vi "Create Events Table_Beltwatch.vi"() -> ()   [LabVIEW 2017, in "Copy of Beltwatch SQLite.lvlib"]
uses:
  Database/Copy of Beltwatch SQLite.lvlib
  Common64/Database/SQ Lite/SQ Lite Cluster Action.ctl
  Beltwatch/SourceCode/BeltWatch Event.ctl
  Beltwatch/SourceCode/BeltWatch Event type.ctl
  Beltwatch/SourceCode/BeltWatch Reading.ctl
  Beltwatch/SourceCode/BeltWatch Alarm Priority.ctl
  Beltwatch/SourceCode/BeltWatch 2D overlay.ctl
  Beltwatch/SourceCode/Overlay mode.ctl
  Beltwatch/SourceCode/Events class.ctl
panel:
  in  "Event":T1={"Position"=17279.321740347055, "Event Type"=enum."Splice", "Area"=261.6138488586849, "Channels"=4503599627369984, "Start position"=17276.619140625, "End  position"=17282.02434006911, "Name"="", "Offset"=0.0, "Length"=1987.8302132084298, "Action marker"="", "Event"=array672x65[43680 elements], "# Defects"=137, "jpg Image"="ASD", "chan maxs"=[0.0, 0.0, 0.0, 0.0, 0.0, 0.0, 0.0, 0.0, 0.0, 0.768, 1.157, 1.845, 4.443, 7.03, 7.383, 6.949, 6.966, 7.121, 6.212, 5.231, 4.772, 4.836, 4.757, 4.587, 4.548, 4.517, 4.666, 4.782, 5.001, 5.174, 5.371, 5.176, 5.098, 4.922, 4.915, 4.636, 4.584, 4.794, 4.884, 4.908, 4.821, 5.046, 5.03, 5.533, 6.356, 7.56, 5.75, 5.5, 7.87, 6.962, 6.495, 1.517, 0.0, 0.0, 0.0, 0.0, 0.0, 0.0, 0.0, 0.0, 0.0, 0.0, 0.0, 0.0], "chan mins"=[0.0, 0.0, 0.0, 0.0, 0.0, 0.0, 0.0, 0.0, 0.0, -1.193, -1.906, -3.257, -6.752, -6.705, -5.152, -4.988, -4.848, -4.552, -4.04, -3.624, -3.41, -3.38, -3.179, -3.134, -3.041, -3.144, -3.022, -3.138, -3.276, -3.433, -3.191, -3.066, -3.021, -2.965, -2.907, -2.884, -2.847, -3.026, -3.293, -3.238, -3.475, -3.528, -3.781, -3.92, -4.795, -6.373, -3.84, -4.344, -6.783, -6.818, -6.448, -1.468, 0.0, 0.0, 0.0, 0.0, 0.0, 0.0, 0.0, 0.0, 0.0, 0.0, 0.0, 0.0], "TimeStamp"=3620638606.9, "Readings"=[{"Reading #"=0, "Readings"=[3.9289019107818604], "Reading Name"="Splice distortion", "Type"=enum."Defect", "Alarm priority"=enum."No Alarm", "Display precision"=0}, {"Reading #"=1, "Readings"=[1328.95654296875], "Reading Name"="Splice length", "Type"=enum."Defect", "Alarm priority"=enum."No Alarm", "Display precision"=0}, {"Reading #"=2, "Readings"=[0.0], "Reading Name"="Splice necking", "Type"=enum."Defect", "Alarm priority"=enum."No Alarm", "Display precision"=0}, {"Reading #"=3, "Readings"=[0.0], "Reading Name"="Splice Max Amplitude ", "Type"=enum."Defect", "Alarm priority"=enum."No Alarm", "Display precision"=0}, {"Reading #"=4, "Readings"=[0.0], "Reading Name"="Width at Splice", "Type"=enum."Defect", "Alarm priority"=enum."No Alarm", "Display precision"=0}, {"Reading #"=5, "Readings"=[0.0], "Reading Name"="Tracking at splice", "Type"=enum."Defect", "Alarm priority"=enum."No Alarm", "Display precision"=0}, {"Reading #"=0, "Readings"=[2.0], "Reading Name"="No. Breaks", "Type"=enum."Defect", "Alarm priority"=enum."No Alarm", "Display precision"=0}, {"Reading #"=1, "Readings"=[7.372896194458008], "Reading Name"="Max  Amplitude (V)", "Type"=enum."Defect", "Alarm priority"=enum."No Alarm", "Display precision"=0}, {"Reading #"=2, "Readings"=[10.810811042785645], "Reading Name"="% Belt Width", "Type"=enum."Defect", "Alarm priority"=enum."No Alarm", "Display precision"=0}, {"Reading #"=3, "Readings"=[0.0], "Reading Name"="% Center Width (%)", "Type"=enum."Defect", "Alarm priority"=enum."No Alarm", "Display precision"=0}, {"Reading #"=4, "Readings"=[0.0], "Reading Name"=" % Max Edge Width", "Type"=enum."Defect", "Alarm priority"=enum."No Alarm", "Display precision"=0}], "ID"=2754970069, "New"=FALSE, "Hires Track"=array672x3[2016 elements], "2D overlay"=[{"group"=[{"X Out"=[1.1431535, 1.1364423, 1.127946, 1.1181517, 1.1072357, 1.0956326, 1.0842199, 1.0731843, 1.0618212, 1.0499833, 1.0380819, 1.0261621, 1.0141459, 1.0021335, 0.990249, 0.9785226, 0.9667934, 0.9549859, 0.9433727, 0.9321445, 0.9210712, 0.909718, 0.8976863, 0.8850422, 0.8726231, 0.8613366, 0.85129416, 0.84175557, 0.8317911, 0.82107306, 0.80985045, 0.79857224, 0.7876048, 0.77725023, 0.76879144, 0.76415265, 0.7633842, 0.7641389, 0.7641741], "Y Out"=[0.40625, 0.4375, 0.46875, 0.5, 0.53125, 0.5625, 0.59375, 0.625, 0.65625, 0.6875, 0.71875, 0.75, 0.78125, 0.8125, 0.84375, 0.875, 0.90625, 0.9375, 0.96875, 1.0, 1.03125, 1.0625, 1.09375, 1.125, 1.15625, 1.1875, 1.21875, 1.25, 1.28125, 1.3125, 1.34375, 1.375, 1.40625, 1.4375, 1.46875, 1.5, 1.53125, 1.5625, 1.59375]}], "Color "=16711680, "Mode"=enum."Line"}, {"group"=[{"X Out"=[1.144922, 1.1339688, 1.1230156, 1.1120626, 1.1011094, 1.0901562, 1.0792031, 1.06825, 1.0572968, 1.0463436, 1.0353905, 1.0244373, 1.0134841, 1.002531, 0.99157786, 0.98062474, 0.96967155, 0.9587184, 0.94776523, 0.9368121, 0.925859, 0.9149058, 0.90395266, 0.89299953, 0.88204634, 0.8710932, 0.86014, 0.8491869, 0.83823377, 0.8272806, 0.81632745, 0.80537426, 0.79442114, 0.783468, 0.7725148, 0.7615617, 0.75060856, 0.7396554, 0.72870225], "Y Out"=[0.40625, 0.4375, 0.46875, 0.5, 0.53125, 0.5625, 0.59375, 0.625, 0.65625, 0.6875, 0.71875, 0.75, 0.78125, 0.8125, 0.84375, 0.875, 0.90625, 0.9375, 0.96875, 1.0, 1.03125, 1.0625, 1.09375, 1.125, 1.15625, 1.1875, 1.21875, 1.25, 1.28125, 1.3125, 1.34375, 1.375, 1.40625, 1.4375, 1.46875, 1.5, 1.53125, 1.5625, 1.59375]}], "Color "=6618880, "Mode"=enum."Line"}, {"group"=[{"X Out"=[1.8756652, 1.8688927, 1.859341, 1.848455, 1.838679, 1.8297793, 1.8196244, 1.8080461, 1.7966759, 1.7862864, 1.7759557, 1.7647399, 1.7527764, 1.7405266, 1.7283434, 1.7166883, 1.7059686, 1.6960664, 1.686259, 1.6760231, 1.6652597, 1.6537125, 1.6410868, 1.627567, 1.6140205, 1.6013763, 1.5898267, 1.5787398, 1.5671003, 1.5549228, 1.5439305, 1.535136, 1.5267466, 1.5169554, 1.507604, 1.5030762, 1.5055563, 1.5104653, 1.5101554], "Y Out"=[0.40625, 0.4375, 0.46875, 0.5, 0.53125, 0.5625, 0.59375, 0.625, 0.65625, 0.6875, 0.71875, 0.75, 0.78125, 0.8125, 0.84375, 0.875, 0.90625, 0.9375, 0.96875, 1.0, 1.03125, 1.0625, 1.09375, 1.125, 1.15625, 1.1875, 1.21875, 1.25, 1.28125, 1.3125, 1.34375, 1.375, 1.40625, 1.4375, 1.46875, 1.5, 1.53125, 1.5625, 1.59375]}], "Color "=16711680, "Mode"=enum."Line"}, {"group"=[{"X Out"=[1.8790404, 1.8683056, 1.8575706, 1.8468357, 1.8361009, 1.825366, 1.8146311, 1.8038963, 1.7931614, 1.7824265, 1.7716916, 1.7609568, 1.7502218, 1.7394869, 1.7287521, 1.7180172, 1.7072823, 1.6965475, 1.6858126, 1.6750777, 1.6643429, 1.653608, 1.642873, 1.6321381, 1.6214033, 1.6106684, 1.5999335, 1.5891987, 1.5784638, 1.5677289, 1.5569941, 1.5462592, 1.5355242, 1.5247893, 1.5140545, 1.5033196, 1.4925847, 1.4818499, 1.471115], "Y Out"=[0.40625, 0.4375, 0.46875, 0.5, 0.53125, 0.5625, 0.59375, 0.625, 0.65625, 0.6875, 0.71875, 0.75, 0.78125, 0.8125, 0.84375, 0.875, 0.90625, 0.9375, 0.96875, 1.0, 1.03125, 1.0625, 1.09375, 1.125, 1.15625, 1.1875, 1.21875, 1.25, 1.28125, 1.3125, 1.34375, 1.375, 1.40625, 1.4375, 1.46875, 1.5, 1.53125, 1.5625, 1.59375]}], "Color "=6618880, "Mode"=enum."Line"}, {"group"=[{"X Out"=[2.474482, 2.4683018, 2.4580495, 2.4460716, 2.4337676, 2.4210174, 2.4081779, 2.3957546, 2.3835855, 2.371664, 2.360103, 2.3485243, 2.3367019, 2.32491, 2.3134542, 2.3026762, 2.2927556, 2.2830057, 2.2726293, 2.262022, 2.2517924, 2.2415245, 2.2306695, 2.2193754, 2.2081182, 2.197146, 2.1865563, 2.1765766, 2.1669314, 2.156789, 2.1457903, 2.1341538, 2.1224358, 2.1115074, 2.1018374, 2.0934274, 2.0864358, 2.080968, 2.0776985, 2.078398], "Y Out"=[0.375, 0.40625, 0.4375, 0.46875, 0.5, 0.53125, 0.5625, 0.59375, 0.625, 0.65625, 0.6875, 0.71875, 0.75, 0.78125, 0.8125, 0.84375, 0.875, 0.90625, 0.9375, 0.96875, 1.0, 1.03125, 1.0625, 1.09375, 1.125, 1.15625, 1.1875, 1.21875, 1.25, 1.28125, 1.3125, 1.34375, 1.375, 1.40625, 1.4375, 1.46875, 1.5, 1.53125, 1.5625, 1.59375]}], "Color "=16711680, "Mode"=enum."Line"}, {"group"=[{"X Out"=[2.4696484, 2.4589303, 2.4482121, 2.437494, 2.4267757, 2.4160576, 2.4053395, 2.3946214, 2.3839033, 2.3731852, 2.362467, 2.351749, 2.3410306, 2.3303125, 2.3195944, 2.3088763, 2.2981582, 2.28744, 2.276722, 2.2660036, 2.2552855, 2.2445674, 2.2338493, 2.2231312, 2.212413, 2.201695, 2.1909766, 2.1802585, 2.1695404, 2.1588223, 2.1481042, 2.137386, 2.126668, 2.1159499, 2.1052315, 2.0945134, 2.0837953, 2.0730772, 2.062359, 2.051641], "Y Out"=[0.375, 0.40625, 0.4375, 0.46875, 0.5, 0.53125, 0.5625, 0.59375, 0.625, 0.65625, 0.6875, 0.71875, 0.75, 0.78125, 0.8125, 0.84375, 0.875, 0.90625, 0.9375, 0.96875, 1.0, 1.03125, 1.0625, 1.09375, 1.125, 1.15625, 1.1875, 1.21875, 1.25, 1.28125, 1.3125, 1.34375, 1.375, 1.40625, 1.4375, 1.46875, 1.5, 1.53125, 1.5625, 1.59375]}], "Color "=6618880, "Mode"=enum."Line"}, {"group"=[{"X Out"=[1.7447797, 1.7451751, 1.741319, 1.7346371, 1.7244854, 1.7100781, 1.6942157, 1.6798319, 1.6669112, 1.6542252, 1.6415849, 1.6298665, 1.6191487, 1.6083951, 1.5975679, 1.5876111, 1.5781267, 1.5678036, 1.5566093, 1.5451726, 1.5332894, 1.5207548, 1.5084059, 1.4974245, 1.4880521, 1.4792299, 1.4697143, 1.4593418, 1.4490005, 1.4395406, 1.4302719, 1.418966, 1.4053056, 1.3919517, 1.3801312, 1.369776, 1.3635503, 1.3650829], "Y Out"=[0.40625, 0.4375, 0.46875, 0.5, 0.53125, 0.5625, 0.59375, 0.625, 0.65625, 0.6875, 0.71875, 0.75, 0.78125, 0.8125, 0.84375, 0.875, 0.90625, 0.9375, 0.96875, 1.0, 1.03125, 1.0625, 1.09375, 1.125, 1.15625, 1.1875, 1.21875, 1.25, 1.28125, 1.3125, 1.34375, 1.375, 1.40625, 1.4375, 1.46875, 1.5, 1.53125, 1.5625]}], "Color "=16711680, "Mode"=enum."Line"}, {"group"=[{"X Out"=[1.7556474, 1.7446698, 1.7336922, 1.7227145, 1.7117369, 1.7007593, 1.6897817, 1.678804, 1.6678264, 1.6568488, 1.6458712, 1.6348935, 1.6239159, 1.6129383, 1.6019607, 1.590983, 1.5800055, 1.5690279, 1.5580503, 1.5470726, 1.536095, 1.5251174, 1.5141398, 1.5031621, 1.4921845, 1.4812069, 1.4702293, 1.4592516, 1.448274, 1.4372964, 1.4263188, 1.4153411, 1.4043636, 1.393386, 1.3824084, 1.3714308, 1.3604531, 1.3494755], "Y Out"=[0.40625, 0.4375, 0.46875, 0.5, 0.53125, 0.5625, 0.59375, 0.625, 0.65625, 0.6875, 0.71875, 0.75, 0.78125, 0.8125, 0.84375, 0.875, 0.90625, 0.9375, 0.96875, 1.0, 1.03125, 1.0625, 1.09375, 1.125, 1.15625, 1.1875, 1.21875, 1.25, 1.28125, 1.3125, 1.34375, 1.375, 1.40625, 1.4375, 1.46875, 1.5, 1.53125, 1.5625]}], "Color "=6618880, "Mode"=enum."Line"}, {"group"=[{"X Out"=[4.364139, 4.46226, 4.364139, 4.46226], "Y Out"=[1.384375, 1.384375, 1.446875, 1.446875]}], "Color "=16727850, "Mode"=enum."Oval"}, {"group"=[{"X Out"=[2.1874433, 2.1874433, 2.1874433, 2.1874433], "Y Out"=[1.5, 1.5, 1.53125, 1.53125]}], "Color "=16727850, "Mode"=enum."Oval"}], "update"=FALSE, "Field #"=0, "Events Class"=enum."Reference", "Sync"=FALSE, "Insert Offset"=0.0, "Next trend"=0.0, "Speed"=0.0}
  out "source":string
  in  "Pre String":string="DROP TABLE IF EXISTS events;\n\n\nCREATE TABLE events (\n  db_id INTEGER PRIMARY KEY AUTOINCREMENT"
  in  "Readingse":T8[](array[typedef])=[{"Include"=TRUE, "Name"="Reading #", "SQLite3 type"=enum."SQLITE_INTEGER"}, {"Include"=TRUE, "Name"="Readings", "SQLite3 type"=enum."SQLITE3_TEXT"}, {"Include"=TRUE, "Name"="Reading Name", "SQLite3 type"=enum."SQLITE3_TEXT"}, {"Include"=TRUE, "Name"="TypeVal", "SQLite3 type"=enum."SQLITE_INTEGER"}, {"Include"=TRUE, "Name"="Alarm priority", "SQLite3 type"=enum."SQLITE_INTEGER"}, {"Include"=FALSE, "Name"="Display precision", "SQLite3 type"=enum."undefined type (0)"}, {"Include"=TRUE, "Name"="TypeStr", "SQLite3 type"=enum."SQLITE3_TEXT"}, {"Include"=TRUE, "Name"="AlarmPriorityStr", "SQLite3 type"=enum."SQLITE3_TEXT"}]
  out "?":errorcluster
  out "String":string
  out "SQLite3 type":T9(ring)
  in  "Events":T8[](array[typedef])=[{"Include"=TRUE, "Name"="Position", "SQLite3 type"=enum."SQLITE_INTEGER"}, {"Include"=TRUE, "Name"="Event Type", "SQLite3 type"=enum."SQLITE_INTEGER"}, {"Include"=TRUE, "Name"="Area", "SQLite3 type"=enum."SQLITE_INTEGER"}, {"Include"=TRUE, "Name"="Channels", "SQLite3 type"=enum."SQLITE_INTEGER"}, {"Include"=TRUE, "Name"="Start position", "SQLite3 type"=enum."SQLITE_INTEGER"}, {"Include"=TRUE, "Name"="End  position", "SQLite3 type"=enum."SQLITE_INTEGER"}, {"Include"=TRUE, "Name"="Name", "SQLite3 type"=enum."SQLITE3_TEXT"}, {"Include"=TRUE, "Name"="Offset", "SQLite3 type"=enum."SQLITE_INTEGER"}, {"Include"=TRUE, "Name"="Length", "SQLite3 type"=enum."SQLITE_INTEGER"}, {"Include"=TRUE, "Name"="Action marker", "SQLite3 type"=enum."SQLITE3_TEXT"}, {"Include"=FALSE, "Name"="Event", "SQLite3 type"=enum."SQLITE_INTEGER"}, {"Include"=TRUE, "Name"="# Defects", "SQLite3 type"=enum."SQLITE_INTEGER"}, {"Include"=TRUE, "Name"="jpg Image", "SQLite3 type"=enum."SQLITE_BLOB"}, {"Include"=FALSE, "Name"="chan maxs", "SQLite3 type"=enum."SQLITE_INTEGER"}, {"Include"=FALSE, "Name"="chan mins", "SQLite3 type"=enum."SQLITE_INTEGER"}, {"Include"=TRUE, "Name"="TimeStamp", "SQLite3 type"=enum."SQLITE_INTEGER"}, {"Include"=TRUE, "Name"="Readings", "SQLite3 type"=enum."SQLITE_INTEGER"}, {"Include"=TRUE, "Name"="ID", "SQLite3 type"=enum."SQLITE_INTEGER"}, {"Include"=TRUE, "Name"="New", "SQLite3 type"=enum."SQLITE_INTEGER"}, {"Include"=TRUE, "Name"="Hires Track", "SQLite3 type"=enum."SQLITE_INTEGER"}, {"Include"=FALSE, "Name"="2D overlay", "SQLite3 type"=enum."SQLITE_INTEGER"}, {"Include"=FALSE, "Name"="update", "SQLite3 type"=enum."SQLITE_INTEGER"}, {"Include"=TRUE, "Name"="Field #", "SQLite3 type"=enum."SQLITE_INTEGER"}, {"Include"=TRUE, "Name"="Events Class", "SQLite3 type"=enum."SQLITE_INTEGER"}, {"Include"=TRUE, "Name"="Sync", "SQLite3 type"=enum."SQLITE_INTEGER"}, {"Include"=TRUE, "Name"="Insert Offset", "SQLite3 type"=enum."SQLITE_INTEGER"}, {"Include"=TRUE, "Name"="Next trend", "SQLite3 type"=enum."SQLITE_INTEGER"}, {"Include"=TRUE, "Name"="Speed", "SQLite3 type"=enum."SQLITE_INTEGER"}]
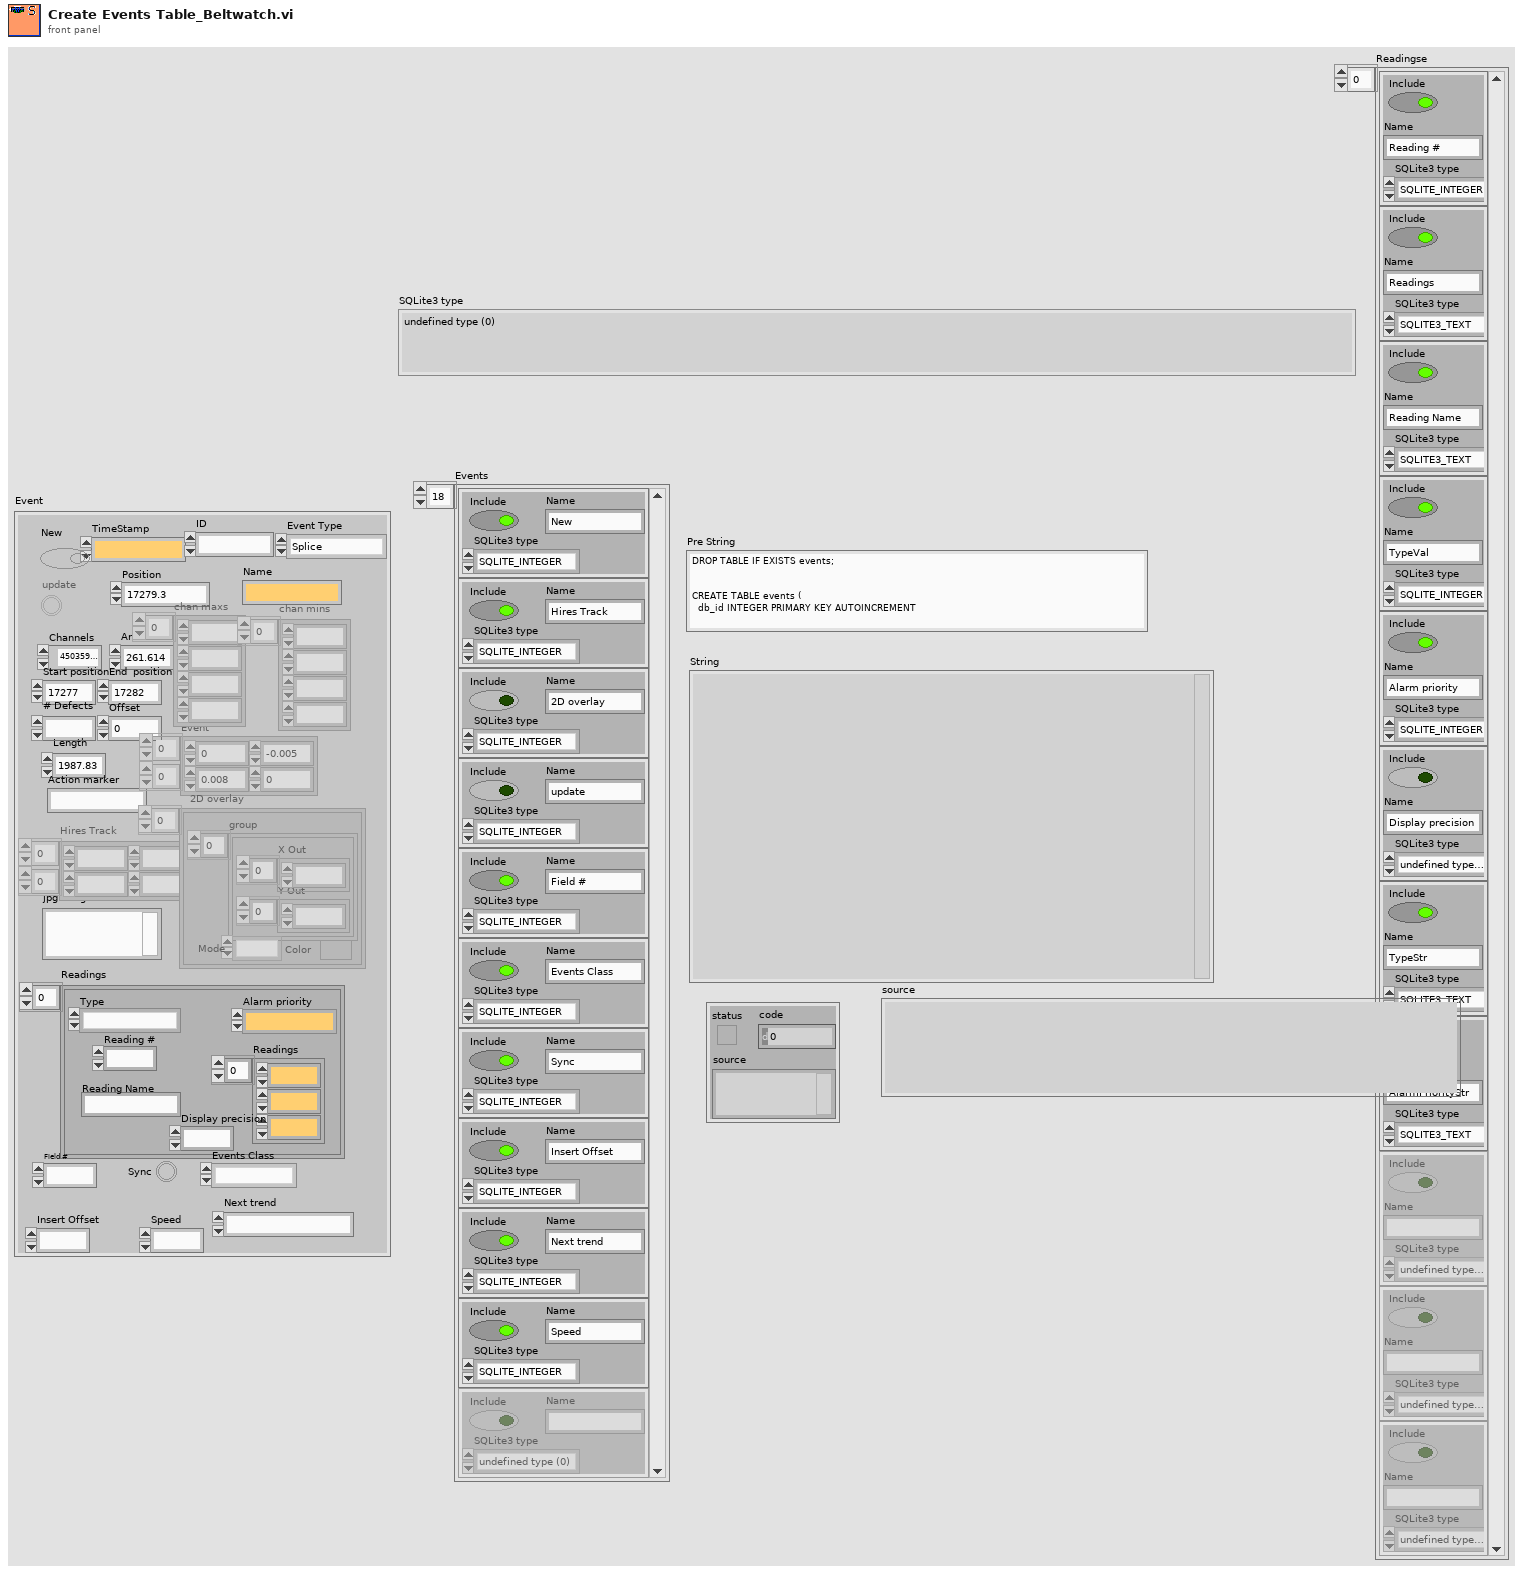
[diagram p1: front panel]
types:
  T1 = typedef "BeltWatch Event.ctl" = cluster{"Position":dbl, "Event Type":T2, "Area":dbl, "Channels":u64, "Start position":dbl, "End  position":dbl, "Name":string, "Offset":dbl, "Length":dbl, "Action marker":string, "Event":dbl[][], "# Defects":i32, "jpg Image":string, "chan maxs":dbl[], "chan mins":dbl[], "TimeStamp":dbl, "Readings":T3[], "ID":u32, "New":bool, "Hires Track":dbl[][], "2D overlay":T5, "update":bool, "Field #":i32, "Events Class":T7, "Sync":bool, "Insert Offset":dbl, "Next trend":dbl, "Speed":dbl}
  T2 = typedef "BeltWatch Event type.ctl" = enum16{"Defect", "Splice", "Break", "Rip", "Track", "Segment", "Belt", "New Splice", "Missing Splice", "None", "Free"}
  T3 = typedef "BeltWatch Reading.ctl" = cluster{"Reading #":i32, "Readings":dbl[], "Reading Name":string, "Type":T2, "Alarm priority":T4, "Display precision":i32}
  T4 = typedef "BeltWatch Alarm Priority.ctl" = enum16{"No Alarm", "High", "Medium", "Low"}
  T5 = typedef "BeltWatch 2D overlay.ctl" = cluster{"group":cluster{"X Out":sgl[], "Y Out":sgl[]}[], "Color ":u32, "Mode":T6}[]
  T6 = typedef "Overlay mode.ctl" = enum16{"Line", "point", "Box", "Oval", "Numbannotation"}
  T7 = typedef "Events class.ctl" = enum16{"Reference", "Inspection", "New", "Tramp", "Align", "Ready"}
  T8 = typedef "Copy of Beltwatch SQLite.lvlib/SQ Lite Cluster Action.ctl" = cluster{"Include":bool, "Name":string, "SQLite3 type":enum32{"undefined type (0)", "SQLITE_INTEGER", "SQLITE_FLOAT", "SQLITE3_TEXT", "SQLITE_BLOB", "SQLITE_NULL", "undefined type", "FloatArray"}}
  T9 = enum32{"undefined type (0)", "SQLITE_INTEGER", "SQLITE_FLOAT", "SQLITE3_TEXT", "SQLITE_BLOB", "SQLITE_NULL", "undefined type"}
  T10 = enum32{"undefined type (0)", "SQLITE_INTEGER", "SQLITE_FLOAT", "SQLITE3_TEXT", "SQLITE_BLOB", "SQLITE_NULL", "undefined type", "FloatArray"}
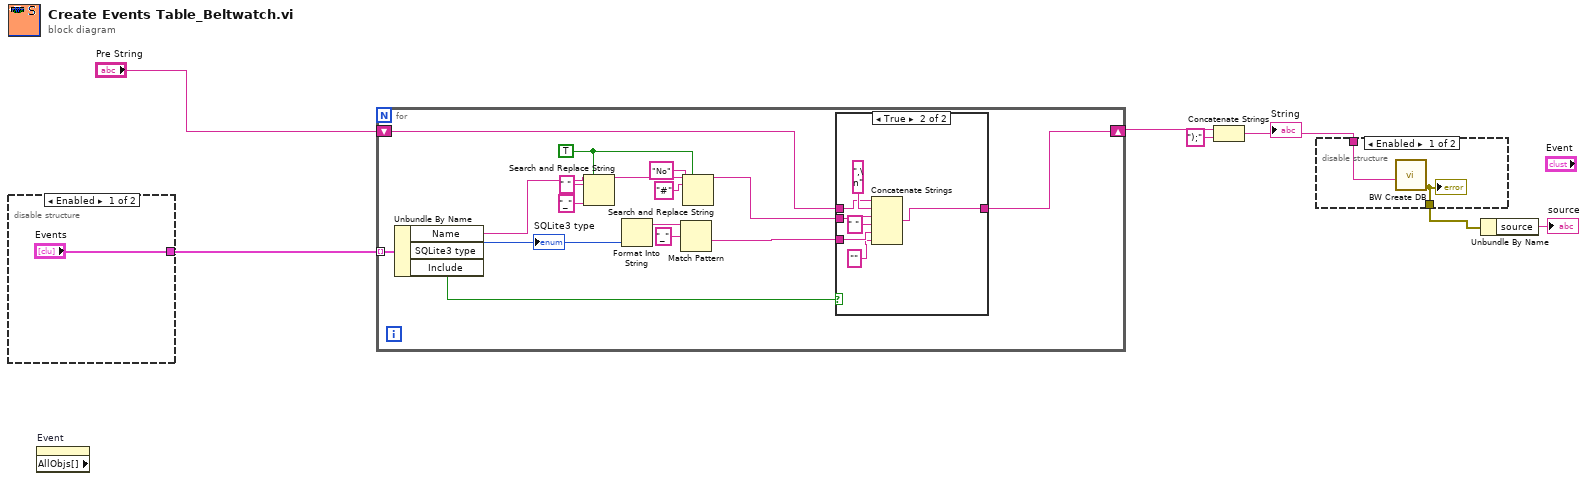
[diagram p0: block diagram]
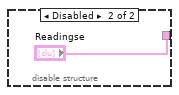
[diagram p2: hidden frame]
diagram:
  n1 = disable-structure shown="Enabled" {
    disable-tunnel: ["Events" "Readingse"] -> w6
    frame Enabled {
    }
    frame Disabled {
    }
  }
  n2 = property on="Event" class="Clust (strict)" props=["AllObjs[]"]() -> ()  [unwired: 2 in, 3 out]
  n3 = for {
    shift-right: [w18] -> w5
    shift-left: "Pre String" -> [w25]
    tunnel: w6 -> [w24] mode=indexing
    w14 = TRUE ("replace all? (F)")
    n4 = Unbundle By Name(w24) -> ("Name"=w17:string, "SQLite3 type"=w22:T10, "Include"=w23:bool)
    "SQLite3 type" <- w22
    n5 = Search and Replace String(replace all?=w14, input string=w17, search string=" ", replace string="_" ("replace string (\"\")")) -> (result string=w13:string)  [unwired: 4 in, 3 out]
    n6 = Format Into String(w22) -> (resulting string=w21:string)  [unwired: 3 in, 1 out]
    n7 = Match Pattern(string=w21, regular expression="_") -> (after substring=w19:string)  [unwired: 1 in, 3 out]
    n8 = Search and Replace String(replace all?=w14, input string=w13, search string="#" ("replace string (\"\")"), replace string="No" ("replace string (\"\")")) -> (result string=w10:string)  [unwired: 4 in, 3 out]
    n9 = case shown="True" w23 {
      tunnel: w25 -> [w26 w28]
      tunnel: w10 -> [_ w33]
      tunnel: w19 -> [_ w31]
      tunnel: [w26 w30] -> w18
      frame False {
      }
      frame True {
        n10 = Concatenate Strings(w28, ",\n" ("string"), w33, " " ("string"), w31, "" ("string")) -> (w30:string)
      }
    }
  }
  n11 = Concatenate Strings(w5, ");" ("string")) -> (w3:string)
  "String" <- w3
  n12 = disable-structure shown="Enabled" {
    disable-tunnel: w3 -> [w35 _]
    disable-tunnel: [w34 _] -> w2
    frame Enabled {
      n13 = call "BW Create DB.vi"("String"=w35) -> ("error out"=w34:errorcluster)  [unwired: 10 in]
      "?" <- w34
    }
    frame Disabled {
    }
  }
  n14 = Unbundle By Name(w2) -> ("source"=→"source":string)
